vi "Spawn Child placeholder.vi"(11 "TEMPLATE Actor in":refnum<class "TEMPLATE Actor.lvclass">) -> (0 "Error out":errorcluster, 3 "TEMPLATE Actor out":refnum<class "TEMPLATE Actor.lvclass">)   [LabVIEW 2020, in "_Template.lvlib" / "Templates.lvlib" / "TEMPLATE jettl Actor.lvlib" / "TEMPLATE Actor.lvlib" / "TEMPLATE Actor.lvclass"]
uses:
  TEMPLATE Actor.lvclass
  C:/git/jettl/src/jettl/jettl/Actor/Actor.lvclass
  jettl/jettl/Actor/Actor.lvclass
  Child UIDs.ctl
  jettl/jettl/Spawn/Async Child.vi
  jettl/jettl/Spawn/Spawn.lvlib
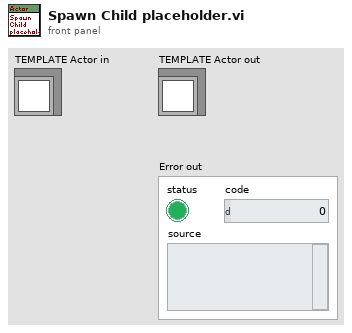
[diagram p1: front panel]
types:
  T1 = typedef "_Template.lvlib/Templates.lvlib/TEMPLATE jettl Actor.lvlib/TEMPLATE Actor.lvlib/TEMPLATE Actor.lvclass/Child UIDs.ctl" = enum16{"placeholder"}
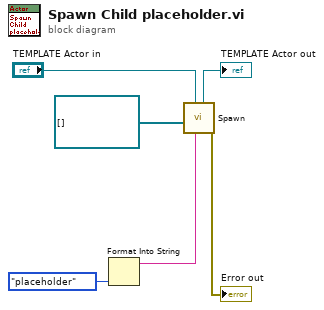
[diagram p0: block diagram]
diagram:
  n1 = Format Into String(Child_UIDs."placeholder" ("Child UIDs")) -> (resulting string=w1:string)  [unwired: 3 in, 1 out]
  n2 = call-poly "Spawn.vi"("UID"=w1, "Actor in"="TEMPLATE Actor in", "Mid Actors"=refnum<class "Actor.lvclass">[] []) -> ("Error out"=→"Error out":errorcluster, "Actor out"=→"TEMPLATE Actor out":refnum<class "TEMPLATE Actor.lvclass">)  [unwired: 7 in]
